vi "Test Process Config File non existing.vi"(8 "error in (no error)":errorcluster, 11 "Process Test In":refnum<class "Process Test.lvclass">) -> (0 "error out":errorcluster, 3 "Process Test Out":refnum<class "Process Test.lvclass">)   [LabVIEW 2020, in "Process Test.lvclass"]
uses:
  Process Test.lvclass
  C:/Program Files (x86)/National Instruments/LabVIEW 2020/vi.lib/Asteme/LUnit/Test Case.lvclass
  Framework/Process/Process.lvclass
  Framework/Process/Process.lvclass/Process.ctl
  <vilib>/Asteme/LUnit/Test Case.lvclass/Test Case.ctl
  <vilib>/Asteme/LUnit/LUnit Assertion Result.lvclass/LUnit Assertion Result.ctl
  Framework/Process/Public/Lifecycle/Get Lifecycle State.vi
  Framework/Process/Private/SubVIs/Wait for finish.vi
  Framework/Process/Protected/Messaging/Enqueue Message.vi
  Framework/Process/Private/SubVIs/Set Lifecycle State.vi
  <vilib>/Asteme/LUnit/Palette/Fail.vi
  <vilib>/Asteme/LUnit/Palette/Pass.vi
  <vilib>/Asteme/LUnit/Set Assertion Type.vi
  <vilib>/Utility/error.llb/Clear Errors.vi
  <vilib>/Asteme/LUnit/Add test result.vi
  <vilib>/Asteme/LUnit/LUnit Write Passed.vi
  <vilib>/Asteme/LUnit/LUnit Get Test Case.vi
  <vilib>/Asteme/LUnit/Assertion Result/LUnit Get Test Name.vi
  <vilib>/Asteme/LUnit/LUnit Write Message.vi
  <vilib>/Asteme/LUnit/LUnit Write Description.vi
  <vilib>/Asteme/LUnit/LUnit Write Assertion Type.vi
  <vilib>/Asteme/LUnit/Read Test Case Name.vi
  <vilib>/Utility/error.llb/Error Cluster From Error Code.vi
  <vilib>/Asteme/LUnit/LUnit Assertion Result.lvclass
  <vilib>/Asteme/LUnit/Test Case.lvclass
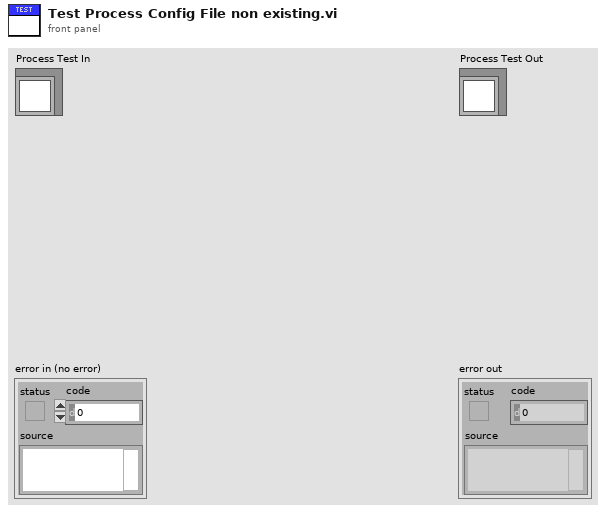
[diagram p1: front panel]
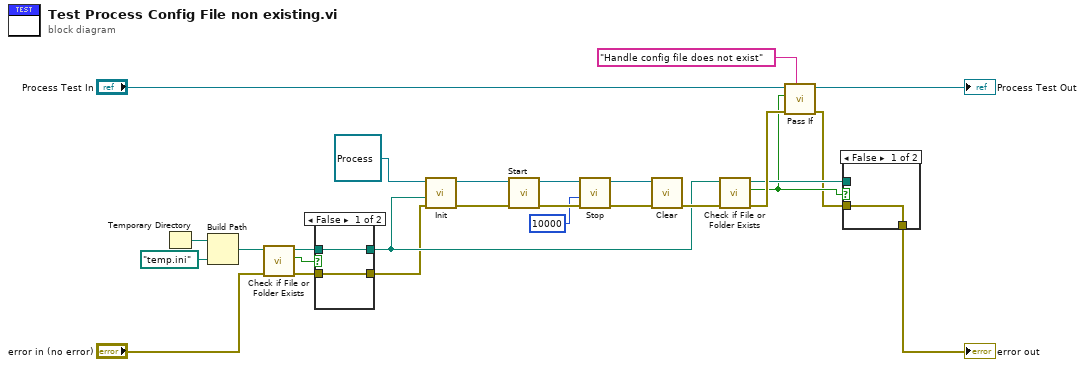
[diagram p0: block diagram]
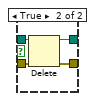
[diagram p2: hidden frame]
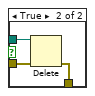
[diagram p3: hidden frame]
diagram:
  n1 = Temporary Directory() -> (w20:path)
  n2 = Build Path(base path=w20, name or relative path=path "temp.ini") -> (appended path=w18:path)
  n3 = call <vilib>:"Check if File or Folder Exists.vi"("error in (no error)"="error in (no error)", "path"=w18) -> ("error out"=w8:errorcluster, "file or folder exists?"=w5:bool, "dup path"=w10:path)  [unwired: 7 in]
  n4 = case shown="False" w5 {
    tunnel: w10 -> [w28 w32]
    tunnel: [w28 w31] -> w9
    tunnel: w8 -> [w27 w30]
    tunnel: [w27 w29] -> w6
    frame False {
    }
    frame True {
      n5 = Delete(path (use dialog)=w32, error in=w30) -> (deleted path=w31:path, error out=w29:errorcluster)  [unwired: 3 in, 1 out]
    }
  }
  n6 = call-dynamic "Init.vi"("error in (no error)"=w6, "Config File Path"=w9, "Process In"=refnum<class "Process.lvclass"> refnum ("Application.lvclass")) -> ("error out"=w23:errorcluster, "Process Out"=w25:refnum<class "Process.lvclass">)  [unwired: 7 in]
  n7 = call "Start.vi"("error in (no error)"=w23, "Process In"=w25) -> ("error out"=w3:errorcluster, "Process Out"=w24:refnum<class "Process.lvclass">)  [unwired: 8 in]
  n8 = call "Stop.vi"("error in (no error)"=w3, "timeout in ms (-1)"=10000, "Process In"=w24) -> ("error out"=w2:errorcluster, "Process Out"=w4:refnum<class "Process.lvclass">)  [unwired: 6 in, 1 out]
  n9 = call-dynamic "Clear.vi"("error in (no error)"=w2, "Process In"=w4) -> ("error out"=w17:errorcluster)  [unwired: 8 in, 1 out]
  n10 = call <vilib>:"Check if File or Folder Exists.vi"("error in (no error)"=w17, "path"=w9) -> ("error out"=w16:errorcluster, "file or folder exists?"=w14:bool, "dup path"=w15:path)  [unwired: 7 in]
  n11 = call <vilib>:"Pass If.vi"("Description"="Handle config file does not exist", "error in (no error)"=w16, "Pass?"=w14, "Test Case In"="Process Test In") -> ("error out"=w13:errorcluster, "Test Case Out"=→"Process Test Out":refnum<class "Process Test.lvclass">)  [unwired: 6 in]
  n12 = case shown="False" w14 {
    tunnel: w15 -> [_ w36]
    tunnel: w13 -> [w33 w35]
    tunnel: [w33 w34] -> w12
    frame False {
    }
    frame True {
      n13 = Delete(path (use dialog)=w36, error in=w35) -> (error out=w34:errorcluster)  [unwired: 3 in, 2 out]
    }
  }
  "error out" <- w12
